vi "HVBuncher.LoadObjects.vi"(0 "i ref in":refnum<vi>, 1 "Objects":string[](array[string]), 3 "ms timeout (10000)":i32=10000, 5 "error in (no error)":errorcluster) -> (14 "i ref out":refnum<vi>, 15 "ObjectsLoaded":string[](array[string]), 17 "timed out":bool, 19 "error out":errorcluster)   [LabVIEW 2014, in "HVBuncher.lvlib"]
doc: "This method loads all requested device objects."
uses:
  HVBuncher.lvlib
  CSCore/CSSystem/CoreDefs/CoreDefs.error_type.ctl
  CSCore/CSSystem/CoreDefs/CoreDefs.error_severity.ctl
  CSCore/CSSystem/CoreLib/CoreLib.string 2 byte array.vi
  CSCore/BaseProcess/BaseProcess.lvlib
  CSCore/CSSystem/CoreLib/CoreLib.lvlib
  CSCore/CSSystem/CSSystemLib/CSSystemLib.lvlib
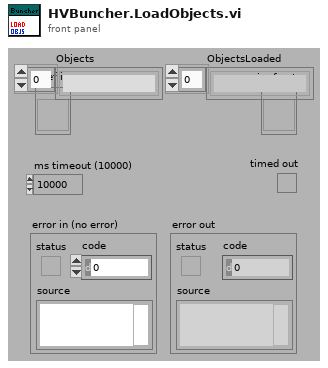
[diagram p1: front panel]
types:
  T1 = typedef "CoreDefs.error_severity.ctl" = enum16{"undefined", "information", "warning", "error", "fatal"}
  T2 = typedef "CoreDefs.error_type.ctl" = enum16{"no error", "can't load process", "can't unload process", "process does not exist", "can't install process", "can't remove process", "unknown function", "time out", "can't execute function", "duplicate queue name", "super not found", "caller queue invalid", "can't ping process", "unknown error", "VISA Error", "VISA timeout", "GPIB timeout", "GPIB error", "communication error", "data type mismatch", "can't read data from OPC server", "can't write data to OPC server", "OET error", "function not implemented", "process already exists", "invalid Shared Variable name", "error writing Shared Variable", "error reading Shared Variable", "invalid client name", "corrupt database", "unknown class", "call not authorized", "parameter out of range", "OET timeout: can't get data to modify", "invalid queue name", "requested operation incompatible with current state", "event undefined", "event disabled", "state undefined", "caller is not a friend", "EventBuilder: bad eventID", "EventBuilder: no DAQ devices", "a thread must not stop itself", "UNUSED ELEMENT4", "DiscArchiver: eventData incomplete", "DiscArchiver: eventData does not belong to run", "DiscArchiver: can't open file", "DiscArchiver: can't write to file", "DiscArchiver: available disc space low", "can't acquire semaphore", "error reading data from database", "notifier object is not existing", "can't register process", "can't unregister process", "illegal event type", "object disabled", "object already exists", "can't change state", "Instrument not found", "no connection to remote node", "invalid reference", "N/A", "UNUSED ELEMENT 1", "element not found", "illegal TCP/IP connection detected", "object does not exist", "invalid access ID", "unknown CS system", "invalid privilige", "unsupported data type", "unsupported server type", "IO server already exists", "Shared Variable already exists"}
  T3 = typedef "CoreDefs.rawDataType.ctl" = i8[]
  T4 = typedef "CoreDefs.call_type.ctl" = cluster{"Object":string, "Selector":string, "CallType":enum16{"simple", "synchronous", "asynchronous"}, "Async Object":string, "Async Selector":string, "Data Descriptor":T5, "Data":T3, "Error #":i32, "Expire":u32}
  T5 = typedef "BaseProcess.lvlib/BaseProcess.descriptor string definition.ctl" = string
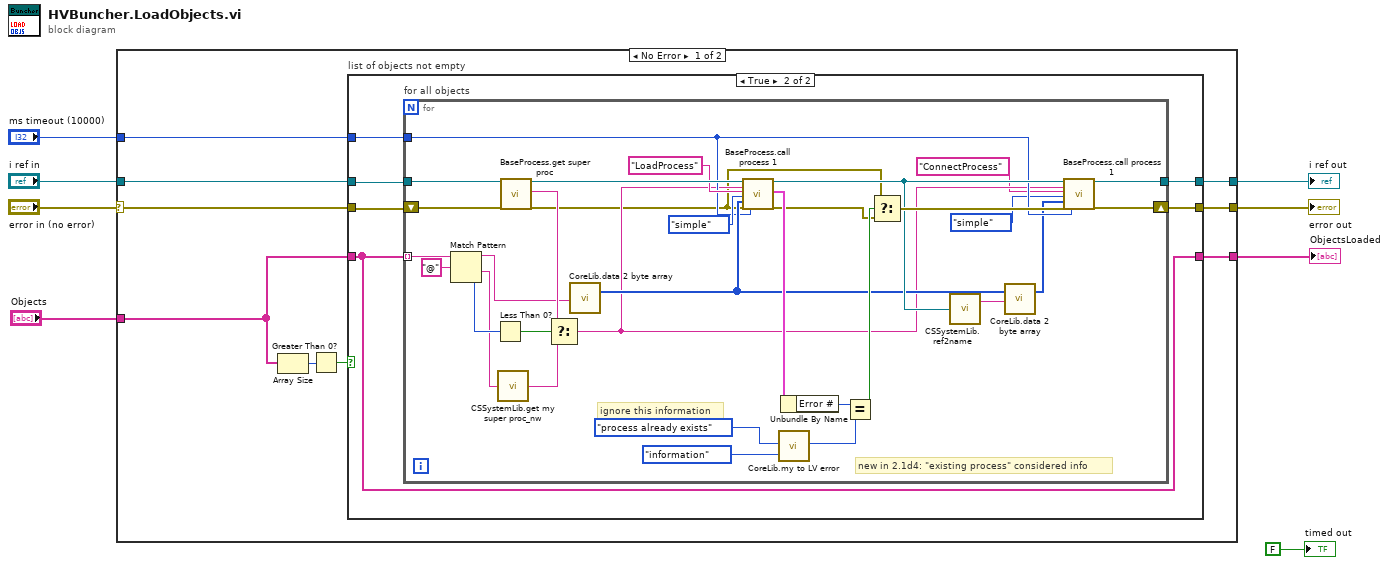
[diagram p0: block diagram]
diagram:
  n1 = case shown="No Error" "error in (no error)" {
    selector: "error in (no error)" -> [w11 w59]
    tunnel: "i ref in" -> [w12 w60]
    tunnel: [w17 w60] -> w7
    tunnel: [w16 w59] -> w5
    tunnel: "ms timeout (10000)" -> [w13 _]
    tunnel: "Objects" -> [w9 _]
    tunnel: [w10 _] -> w1
    frame No Error {
      n2 = Array Size(array=w9) -> (size(s)=w14:i32)
      n3 = Greater Than 0?(x=w14) -> (x > 0?=w15:bool)
      n4 = case "list of objects not empty" shown="True" w15 {
        tunnel: w9 -> [w18 w21]
        tunnel: w12 -> [w20 w23]
        tunnel: [w20 w26] -> w17
        tunnel: w11 -> [w19 w22]
        tunnel: [w19 w25] -> w16
        tunnel: w13 -> [_ w24]
        tunnel: [w18 w21] -> w10
        frame False {
        }
        frame True {
          n5 = for "for all objects" {
            tunnel: w21 -> [w58] mode=indexing
            tunnel: w23 -> [w55]
            tunnel: [w51] -> w26
            shift-right: [w43] -> w25
            shift-left: w22 -> [w50]
            tunnel: w24 -> [w32]
            # "new in 2.1d4: \"existing process\" considered info"
            # "ignore this information"
            n6 = Match Pattern(string=w58, regular expression="@") -> (before substring=w38:string, after substring=w37:string, offset past match=w56:i32)  [unwired: 1 in, 1 out]
            n7 = Less Than 0?(x=w56) -> (x < 0?=w53:bool)
            n8 = call "CSSystemLib.get my super proc_nw.vi"("systemID"=w37) -> ("superProcName"=w36:string)
            n9 = call "BaseProcess.get super proc.vi"("i ref in"=w55, "error in (no error)"=w50) -> ("i ref out"=w54:refnum<vi>, "SuperProc"=w52:string, "error out"=w27:errorcluster)  [unwired: 15 in]
            n10 = Select(t=w52, s=w53, f=w36) -> (s? t:f=w31:string)
            n11 = call-poly "CoreLib.data 2 byte array.vi"("string"=w38) -> ("byteArray out"=w34:T3)  [unwired: 18 in]
            n12 = call "BaseProcess.call process 1.vi"("i ref in"=w54, "Object"=w31, "Selector"="LoadProcess", "CallType"=enum16{"simple", "synchronous", "asynchronous"}."simple", "Data"=w34, "error in (no error)"=w27, "timeout (ms)"=w32) -> ("i ref out"=w41:refnum<vi>, "call cluster out"=w49:T4, "error out"=w44:errorcluster)  [unwired: 10 in]
            n13 = call "CoreLib.my to LV error.vi"("ErrorTypes"=CoreDefs.error_type."process already exists", "severityLevel"=CoreDefs.error_severity."information") -> ("LV error code"=w46:i32)  [unwired: 16 in, 1 out]
            n14 = Unbundle By Name(w49) -> ("Error #"=w48:i32)
            n15 = Equal?(x=w48, y=w46) -> (x = y?=w45:bool)
            n16 = Select(t=w27, s=w45, f=w44) -> (s? t:f=w42:errorcluster)
            n17 = call "CSSystemLib.ref2name.vi"("obj refnum"=w41) -> ("name"=w39:string)
            n18 = call-poly "CoreLib.data 2 byte array.vi"("byteArray"=w34, "string"=w39) -> ("byteArray out"=w28:T3)  [unwired: 17 in]
            n19 = call "BaseProcess.call process 1.vi"("i ref in"=w41, "Object"=w31, "Selector"="ConnectProcess", "CallType"=enum16{"simple", "synchronous", "asynchronous"}."simple", "Data"=w28, "error in (no error)"=w42, "timeout (ms)"=w32) -> ("i ref out"=w51:refnum<vi>, "error out"=w43:errorcluster)  [unwired: 10 in, 1 out]
          }
        }
      }
    }
    frame Error {
    }
  }
  "error out" <- w5
  "i ref out" <- w7
  "ObjectsLoaded" <- w1
  "timed out" <- FALSE ("timed out")
